vi "goldenDiff.vi"(8 "error in (no error)":errorcluster, 10 "Current Image":T1, 11 "Current Test Directory":string) -> (0 "error out":errorcluster, 1 "Report String":string, 2 "Images Same?":bool, 3 "Diff Image Data":T1)   [LabVIEW 2018, in "Image_Diff.lvlib"]
doc: "This VI loads a golden template image from a filepath and diffs it with an input image. This VI returns: (Bool ImagesSame?, Struct_FlattenedImageData DiffImageData, String ReportString)\n\nBool ImagesSame? - Reports whether or not the diff found any discrepancies between the golden image and the input image\n\nStruct_FlattenedImageData DiffImageData - Contains flattened image data which can be used in LabVIEW to display the image showing the differences between the two pictures (highlighted in red)\n\nString ReportString - a pre-formatted HTML string that can be written directly to Step.Result.ReportText in TestStand to add images into the auto-generated Test Report"
uses:
  Image_Diff.lvlib
  <vilib>/picture/picture.llb/imagedata.ctl
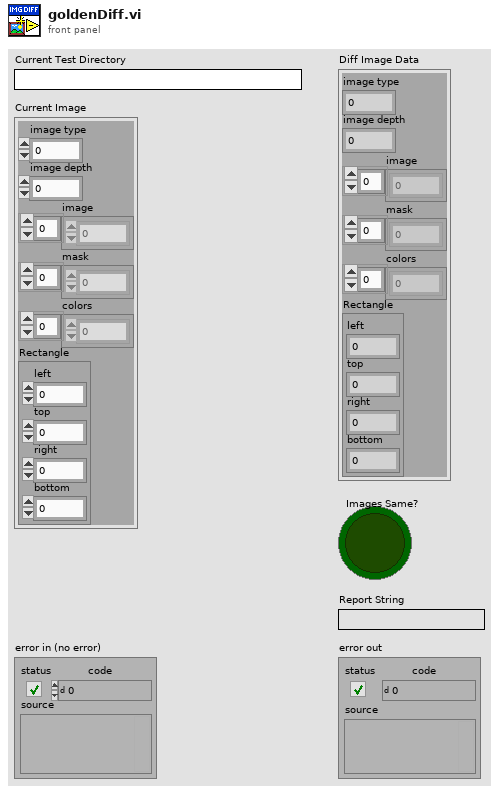
[diagram p1: front panel]
types:
  T1 = typedef "imagedata.ctl" = cluster{"image type":i32, "image depth":i32, "image":u8[], "mask":u8[], "colors":u32[], "Rectangle":cluster{"left":i16, "top":i16, "right":i16, "bottom":i16}}
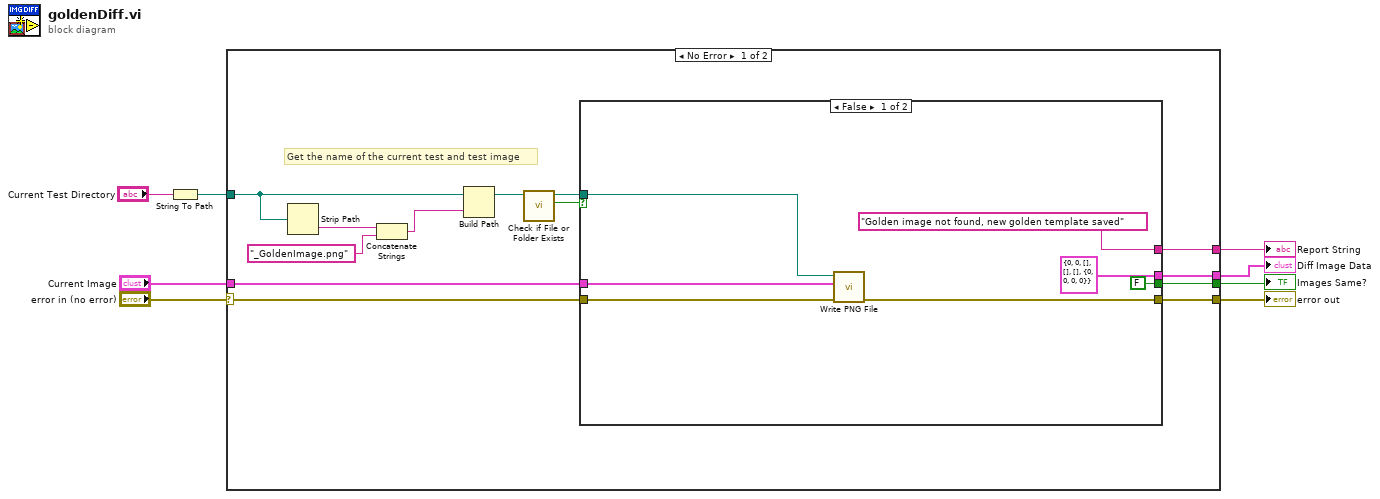
[diagram p0: block diagram]
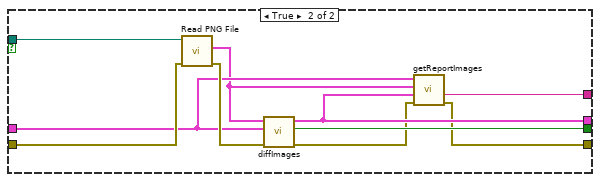
[diagram p2: hidden frame]
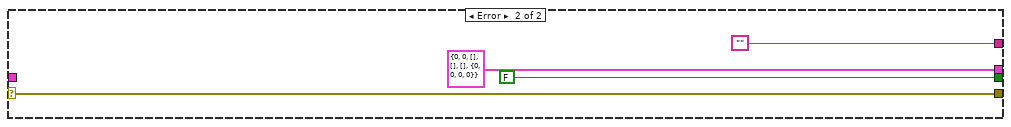
[diagram p3: hidden frame]
diagram:
  n1 = String To Path(string="Current Test Directory") -> (path=w2:path)
  n2 = case shown="No Error" "error in (no error)" {
    selector: "error in (no error)" -> [w20 w40]
    tunnel: [w17 w40] -> w8
    tunnel: [w19 T1 {"image type"=0, "image depth"=0, "image"=[], "mask"=[], "colors"=[], "Rectangle"={"left"=0, "top"=0, "right"=0, "bottom"=0}} ("Diff Image Data")] -> w6
    tunnel: [w21 FALSE ("Differences Found?")] -> w5
    tunnel: "Current Image" -> [w18 _]
    tunnel: w2 -> [w12 _]
    tunnel: [w16 ""] -> w3
    frame No Error {
      # "Get the name of the current test and test image"
      n3 = Strip Path(path=w12) -> (name=w11:string)  [unwired: 1 out]
      n4 = Concatenate Strings(w11, "_GoldenImage.png" ("name or relative path")) -> (w9:string)
      n5 = Build Path(base path=w12, name or relative path=w9) -> (appended path=w13:path)
      n6 = call <vilib>:"Check if File or Folder Exists.vi"("path"=w13) -> ("file or folder exists?"=w15:bool, "dup path"=w14:path)  [unwired: 8 in, 1 out]
      n7 = case shown="False" w15 {
        tunnel: [FALSE ("Differences Found?") w38] -> w21
        tunnel: w14 -> [w22 w37]
        tunnel: w20 -> [w28 w36]
        tunnel: [T1 {"image type"=0, "image depth"=0, "image"=[], "mask"=[], "colors"=[], "Rectangle"={"left"=0, "top"=0, "right"=0, "bottom"=0}} ("Diff Image Data") w34] -> w19
        tunnel: w18 -> [w26 w33]
        tunnel: [w27 w30] -> w17
        tunnel: ["Golden image not found, new golden template saved" ("Report String") w29] -> w16
        frame False {
          n8 = call <vilib>:"Write PNG File.vi"("error in (no error)"=w28, "image data"=w26, "path to PNG file"=w22) -> ("error out"=w27:errorcluster)  [unwired: 7 in, 1 out]
        }
        frame True {
          n9 = call <vilib>:"Read PNG File.vi"("error in (no error)"=w36, "path to PNG file"=w37) -> ("error out"=w35:errorcluster, "image data"=w32:T1)  [unwired: 7 in, 1 out]
          n10 = call "diffImages.vi"("error in (no error)"=w35, "Image 2"=w33, "Image 1"=w32) -> ("error out"=w31:errorcluster, "Images Same?"=w38:bool, "Diff Image Data"=w34:T1)  [unwired: 6 in]
          n11 = call "getReportImages.vi"("error in (no error)"=w31, "Diff Image"=w34, "Golden Image"=w32, "Current Image"=w33) -> ("error out"=w30:errorcluster, "Report String"=w29:string)  [unwired: 6 in]
        }
      }
    }
    frame Error {
    }
  }
  "error out" <- w8
  "Diff Image Data" <- w6
  "Images Same?" <- w5
  "Report String" <- w3
